vi "RN Test.vi"() -> ()   [LabVIEW 2015]
uses:
  <vilib>/Analysis/NI_AALBase.lvlib
panel:
  out "size(s)":i32
  out "Waveform Graph":dbl[][](graph)
  out "XY Graph 2":T1(graph)
  out "XY Graph":T1(graph)
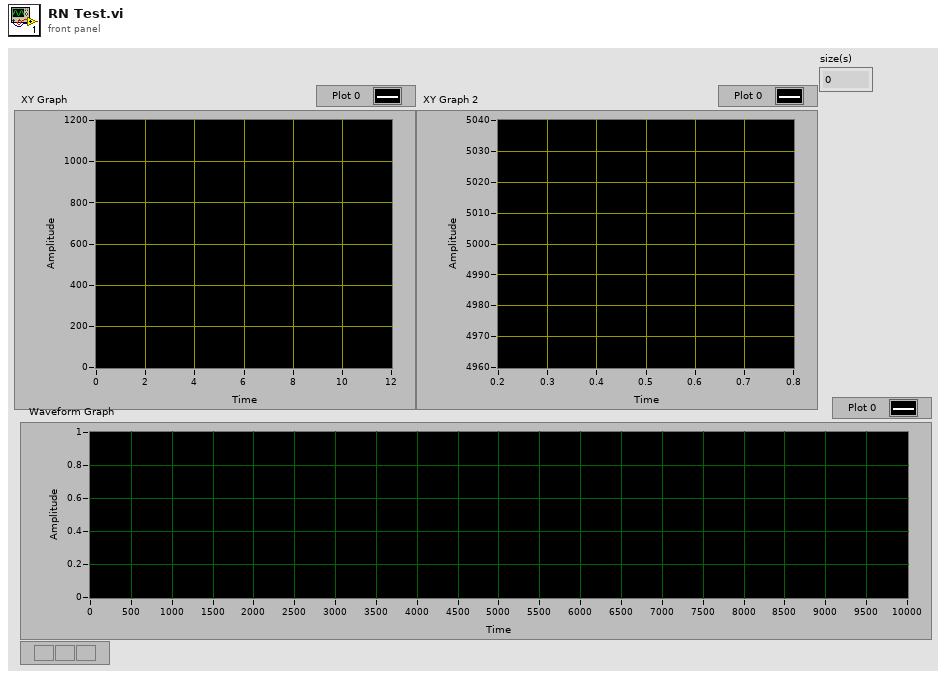
[diagram p1: front panel]
types:
  T1 = cluster{"X Values":dbl[], "Histogram: h(x)":i32[]}
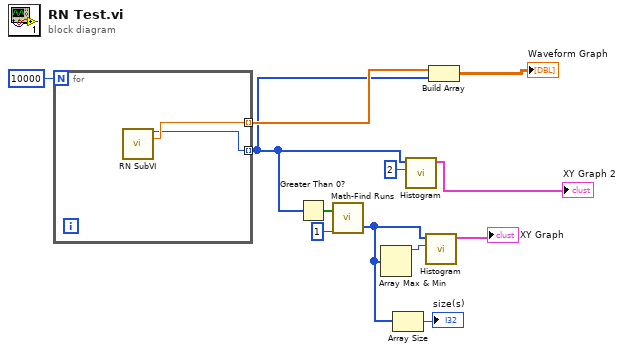
[diagram p0: block diagram]
diagram:
  n1 = for {
    N: 10000 -> [_]
    tunnel: [w14] -> w8 mode=indexing
    tunnel: [w13] -> w5 mode=indexing
    n2 = call "RN SubVI.vi"() -> ("Numeric"=w13:i32, "number: 0 to 1"=w14:dbl)  [unwired: 14 in]
  }
  n3 = Greater Than 0?(x=w5) -> (x > 0?=w6:bool[])
  n4 = call "Math-Find Runs.vi"("Min Run Length"=1, "Array"=w6) -> ("Length"=w2:i32[])  [unwired: 1 out]
  n5 = Array Max & Min(array=w2) -> (max value=w4:i32)  [unwired: 3 out]
  n6 = Array Size(array=w2) -> (size(s)=→"size(s)":i32)
  n7 = call <vilib>:"Histogram.vi"("intervals"=2, "X"=w5) -> ("Histogram Graph"=→"XY Graph 2":T1)  [unwired: 6 in, 3 out]
  n8 = call <vilib>:"Histogram.vi"("intervals"=w4, "X"=w2) -> ("Histogram Graph"=→"XY Graph":T1)  [unwired: 6 in, 3 out]
  n9 = Build Array(w8, w5) -> (→"Waveform Graph":dbl[][])
